vi "Set Initialization Data - FP_Emulator.vi"(8 "error in":errorcluster, 11 "Device Manager in":refnum<class "Device Manager.lvclass">) -> (0 "error out":errorcluster, 3 "Device Manager out":refnum<class "Device Manager.lvclass">)   [LabVIEW 2017, in "Device Manager.lvclass"]
doc: "In this VI you can set the initialization data of a statically-linked subWorker."
uses:
  Device Manager.lvclass
  Front Panel Emulator/Initialization Data.ctl
  Front Panel Emulator/Response Cases.ctl
  <vilib>/addons/_Workers/Library/Case Label.ctl
  Device Manager.lvclass/Device Manager.ctl
  Front Panel Emulator/Front Panel Emulator.lvclass
  C:/Program Files (x86)/National Instruments/LabVIEW 2017/vi.lib/addons/_Workers/Library/Classes/Worker/Worker.lvclass
  <vilib>/addons/_Workers/Library/Workers.lvlib
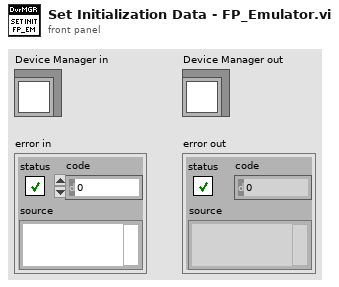
[diagram p1: front panel]
types:
  T1 = typedef "Front Panel Emulator.lvclass/Initialization Data.ctl" = cluster{"Response Cases":T2}
  T2 = typedef "Front Panel Emulator.lvclass/Response Cases.ctl" = cluster{"Set Position":T3}
  T3 = typedef "Workers.lvlib/Case Label.ctl" = string
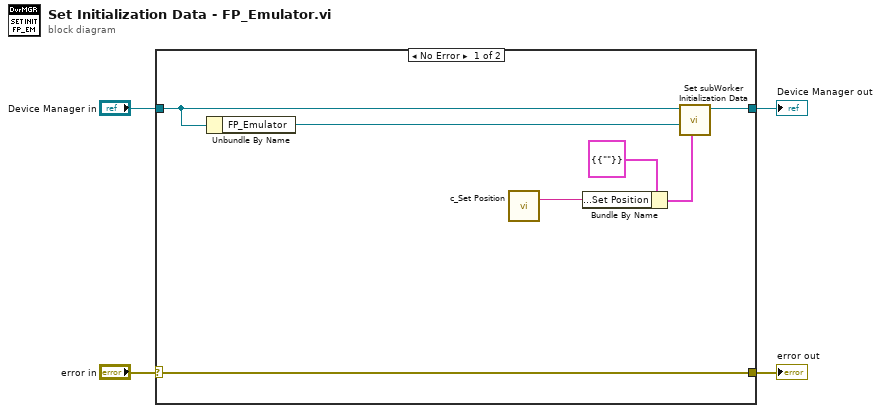
[diagram p0: block diagram]
diagram:
  n1 = case shown="No Error" "error in" {
    selector: "error in" -> [w11 w13]
    tunnel: [w11 w13] -> w3
    tunnel: [w9 w12] -> w2
    tunnel: "Device Manager in" -> [w8 w12]
    frame No Error {
      n2 = Unbundle By Name(w8) -> ("FP_Emulator"=w10:refnum<class "Front Panel Emulator.lvclass">)
      n3 = call "c_Set Position.vi"() -> ("Case Label"=w5:T3)  [unwired: 1 in]
      n4 = Bundle By Name(cluster=T1 {"Response Cases"={"Set Position"=""}} ("Initialization Data"), "Response Cases.Set Position"=w5) -> (w6:T1)
      n5 = call-dynamic "Set subWorker Initialization Data.vi"("Initialization Data"=w6, "subWorker"=w10, "Worker"=w8) -> ("Worker out"=w9:refnum<class "Device Manager.lvclass">)  [unwired: 8 in]
    }
    frame Error {
    }
  }
  "error out" <- w3
  "Device Manager out" <- w2
